vi "unpack_map_len.vi"(3 "error in":errorcluster, 5 "u":u64) -> (0 "error out":errorcluster, 1 "n":u32, 2 "u out":u64)   [LabVIEW 2019, in "msgunpack.lvlib"]
doc: "Begins unpacking a map object from the buffer. Returns the number N of (key,value) pairs in the map list; the user is then resposible for unpacking the next 2*N elements which form this map list."
uses:
  msgunpack.lvlib
  msgpack.lvlib
  msgpackalt.dll
panel:
  # "msgpack"
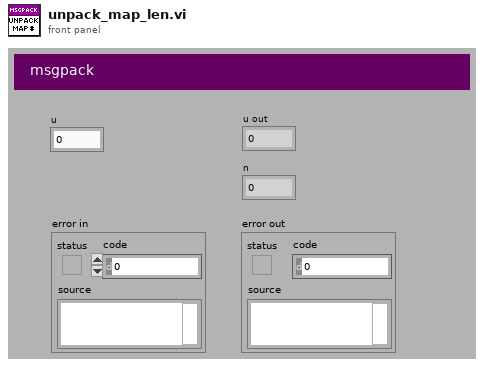
[diagram p1: front panel]
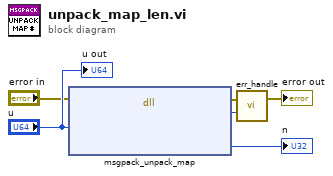
[diagram p0: block diagram]
diagram:
  n1 = dll-call lib="C:/Users/Patrick/Documents/GitHub/Instrument-Framework/lvsrc/SMOs/JSON-RPC-2019/lv-venv/lv.lib/vi.lib/addons/msgpack/msgpackalt.dll" fn="msgpack_unpack_map"(error in="error in", "p"="u") -> (error out=w2:errorcluster, "return type"=w3:i32, "n"=→"n":u32)  [unwired: 4 in, 1 out]
  n2 = call "err_handle.vi"("retval"=w3, "error in"=w2) -> ("error out"=→"error out":errorcluster)  [unwired: 1 in]
  "u out" <- "u"
